vi "Name To Sensor.vi"(10 "Sensor Name":string) -> (0 "Found?":bool, 2 "Sensor Enum":T1)   [LabVIEW 2015]
uses:
  Sensors/Sensor Enum.ctl
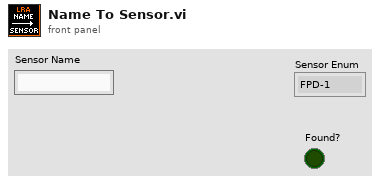
[diagram p1: front panel]
types:
  T1 = typedef "Sensor Enum.ctl" = enum16{"FPD-1", "FPD-2", "FPD-3", "OPD-1", "OPD-2", "OPD-3", "AP-1", "VBAT", "VCOMP", "ICOMP", "TD10"}
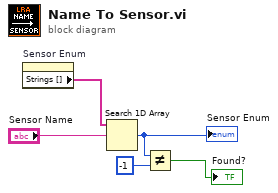
[diagram p0: block diagram]
diagram:
  n1 = property on="Sensor Enum" class="Enum (strict)"() -> ("Strings []"=w5:string[])  [unwired: 2 in, 2 out]
  n2 = Search 1D Array(1D array=w5, element="Sensor Name") -> (index of element=w3:i32)  [unwired: 1 in]
  "Sensor Enum" <- w3
  n3 = Not Equal?(x=w3, y=-1) -> (x != y?=→"Found?":bool)
